vi "Read To String_True.vi"(8 "error in (no error)":errorcluster, 11 "Boolean in":refnum<class "Abs_Boolean.lvclass">) -> (0 "error out":errorcluster, 2 "To String:True":string, 3 "Boolean out":refnum<class "Abs_Boolean.lvclass">)   [LabVIEW 2021, in "Abs_Boolean.lvclass"]
uses:
  Abs_Boolean.lvclass
  Abs_Boolean.lvclass/Abs_Boolean.ctl
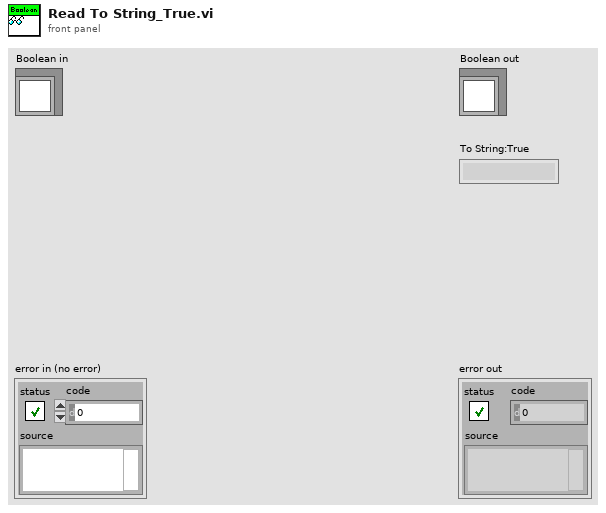
[diagram p1: front panel]
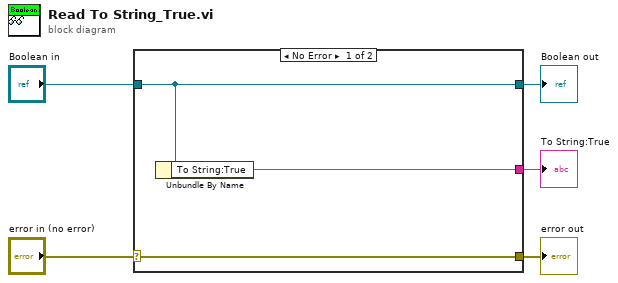
[diagram p0: block diagram]
diagram:
  n1 = case shown="No Error" "error in (no error)" {
    selector: "error in (no error)" -> [w8 w9]
    tunnel: [w8 w9] -> w4
    tunnel: [w7 w10] -> w2
    tunnel: "Boolean in" -> [w7 w10]
    tunnel: [w6 _] -> w1
    frame No Error {
      n2 = Unbundle By Name(w7) -> ("To String:True"=w6:string)
    }
    frame Error {
    }
  }
  "error out" <- w4
  "Boolean out" <- w2
  "To String:True" <- w1
